vi "TrajectoryExecuteRelative.vi"(8 "Init":bool, 10 "End Relative\nOrientation Deg":dbl, 11 "Trajectory":T1 {"States"."POSE"."ROTATION"."SIN" format="%13.4f"; "States"."POSE"."ROTATION"."COS" format="%13.4f"; "States"."POSE"."ROTATION"."VALUE" format="%13.4f"; "States"."POSE"."TRANSLATION"."Y" format="%14.3f"; "States"."POSE"."TRANSLATION"."X" format="%14.3f"; "TotalTImeSecs" format="%20.3f"}) -> (0 "AtReference":bool, 2 "Done":bool, 3 "Chassis Velocity Target Met,Met,Rad":T6 {"vOmega" format="%10.3f"; "vY" format="%10.3f"; "vX" format="%10.3f"})   [LabVIEW 2023]
uses:
  <vilib>/Rock Robotics/WPI/ThirdParty/JAS_Junk/TrajLib/TypeDef/CHASSIS_SPEEDS.ctl
  <vilib>/Rock Robotics/WPI/ThirdParty/JAS_Junk/TrajLib/TypeDef/TRAJECTORY.ctl
  <vilib>/Rock Robotics/WPI/ThirdParty/JAS_Junk/TrajLib/TypeDef/TRAJ_STATE.ctl
  <vilib>/Rock Robotics/WPI/ThirdParty/JAS_Junk/TrajLib/TypeDef/POSE2D.ctl
  <vilib>/Rock Robotics/WPI/ThirdParty/JAS_Junk/TrajLib/TypeDef/TRANSLATION2D.ctl
  <vilib>/Rock Robotics/WPI/ThirdParty/JAS_Junk/TrajLib/TypeDef/ROTATION2D.ctl
  <vilib>/Rock Robotics/WPI/ThirdParty/JAS_Junk/TrajLib/VI/Util_GetTime_U32.vi
  <vilib>/Rock Robotics/WPI/ThirdParty/JAS_Junk/TrajLib/SwerveOdometry_UpdateX.vi
  <vilib>/Rock Robotics/WPI/ThirdParty/JAS_Junk/TrajLib/SwerveOdometry_ResetPosition.vi
  <vilib>/Rock Robotics/WPI/ThirdParty/JAS_Junk/TrajLib/SwerveOdometry_New.vi
  <vilib>/Rock Robotics/WPI/ThirdParty/JAS_Junk/TrajLib/HolDrvCtrl_New.vi
  <vilib>/Rock Robotics/WPI/ThirdParty/JAS_Junk/TrajLib/HolDrvCtrl_PackPID.vi
  <vilib>/Rock Robotics/WPI/ThirdParty/JAS_Junk/TrajLib/HolDrvCtrl_SetTolerance.vi
  <vilib>/Rock Robotics/WPI/ThirdParty/JAS_Junk/TrajLib/HolDrvCtrl_SetEnabled.vi
  <vilib>/Rock Robotics/WPI/ThirdParty/JAS_Junk/TrajLib/HolDrvCtrl_Calculate_Trajectory.vi
  <vilib>/Rock Robotics/WPI/ThirdParty/JAS_Junk/TrajLib/HolDrvCtrl_AtReference.vi
  <vilib>/Rock Robotics/WPI/ThirdParty/JAS_Junk/TrajLib/ProfiledPIDController_NewPeriod.vi
  <vilib>/Rock Robotics/WPI/ThirdParty/JAS_Junk/TrajLib/ProfiledPIDController_SetIntegratorRange.vi
  <vilib>/Rock Robotics/WPI/ThirdParty/JAS_Junk/TrajLib/ProfiledPIDController_DisableContInput.vi
  <vilib>/Rock Robotics/WPI/ThirdParty/JAS_Junk/TrajLib/ProfiledPIDController_EnableContInput.vi
  <vilib>/Rock Robotics/WPI/ThirdParty/JAS_Junk/TrajLib/TrapProfConstraint_New.vi
  <vilib>/Rock Robotics/WPI/ThirdParty/JAS_Junk/TrajLib/Rotation2d_Plus.vi
  <vilib>/Rock Robotics/WPI/ThirdParty/JAS_Junk/TrajLib/Twist2d_Create.vi
  <vilib>/Rock Robotics/WPI/ThirdParty/JAS_Junk/TrajLib/Rotation2d_Minus.vi
  <vilib>/Rock Robotics/WPI/ThirdParty/JAS_Junk/TrajLib/Pose2d_getTranslation.vi
  <vilib>/Rock Robotics/WPI/ThirdParty/JAS_Junk/TrajLib/Pose2d_New_TRRO.vi
  <vilib>/Rock Robotics/WPI/ThirdParty/JAS_Junk/TrajLib/VI/SwerveModulePosition_Get.vi
  <vilib>/Rock Robotics/WPI/ThirdParty/JAS_Junk/TrajLib/VI/SwerveModulePosition_New.vi
  <vilib>/Rock Robotics/WPI/ThirdParty/JAS_Junk/TrajLib/Twist2d_GetAll.vi
  <vilib>/Rock Robotics/WPI/ThirdParty/JAS_Junk/TrajLib/Pose2d_getRotation.vi
  <vilib>/Rock Robotics/SystemInterfaces/NetworkCommunication/NetComm_UsageReport_report.vi
  <vilib>/Rock Robotics/WPI/ThirdParty/JAS_Junk/TrajLib/PIDController_NewPeriod.vi
  <vilib>/Rock Robotics/WPI/ThirdParty/JAS_Junk/TrajLib/PIDController_SetIntegratorRange.vi
  <vilib>/Rock Robotics/WPI/ThirdParty/JAS_Junk/TrajLib/PIDController_Reset.vi
  <vilib>/Rock Robotics/WPI/ThirdParty/JAS_Junk/TrajLib/HolDrvCtrl_Calculate.vi
  <vilib>/Rock Robotics/WPI/ThirdParty/JAS_Junk/TrajLib/Pose2d_getXYAngle.vi
  <vilib>/Rock Robotics/WPI/ThirdParty/JAS_Junk/TrajLib/Rotation2d_GetRadians.vi
  <vilib>/Rock Robotics/WPI/ThirdParty/JAS_Junk/TrajLib/TrapProfState_New.vi
  <vilib>/Rock Robotics/WPI/ThirdParty/JAS_Junk/TrajLib/PIDController_DisableContinousInput.vi
  <vilib>/Rock Robotics/WPI/ThirdParty/JAS_Junk/TrajLib/PIDController_EnableContinousInput.vi
  <vilib>/Rock Robotics/WPI/ThirdParty/JAS_Junk/TrajLib/Rotation2d_RotateBy.vi
  <vilib>/Rock Robotics/WPI/ThirdParty/JAS_Junk/TrajLib/Rotation2d_UnaryMinus.vi
  <vilib>/Rock Robotics/WPI/ThirdParty/JAS_Junk/TrajLib/Rotation2d_GetAngleCosSin.vi
  <vilib>/Rock Robotics/WPI/ThirdParty/JAS_Junk/TrajLib/Pose2d_RelativeTo.vi
  <vilib>/Rock Robotics/WPI/ThirdParty/JAS_Junk/TrajLib/ProfiledPIDController_Calculate_Meas_Goal.vi
  <vilib>/Rock Robotics/WPI/ThirdParty/JAS_Junk/TrajLib/PIDController_Calculate_SP_PV.vi
  <vilib>/Rock Robotics/WPI/ThirdParty/JAS_Junk/TrajLib/ProfiledPIDController_Reset_PosOnly.vi
  <vilib>/Rock Robotics/WPI/ThirdParty/JAS_Junk/TrajLib/ChassisSpeeds_FromFieldRelativeSpeeds.vi
  <vilib>/Rock Robotics/WPI/ThirdParty/JAS_Junk/TrajLib/Rotation2d_CreateXY.vi
  <vilib>/Rock Robotics/WPI/ThirdParty/JAS_Junk/TrajLib/Transform2d_Create_PosePose.vi
  <vilib>/Rock Robotics/WPI/ThirdParty/JAS_Junk/TrajLib/ProfiledPIDController_SetGoal_PosOnly.vi
  <vilib>/Rock Robotics/WPI/ThirdParty/JAS_Junk/TrajLib/ProfiledPIDController_Calculate_Meas.vi
  <vilib>/Rock Robotics/WPI/ThirdParty/JAS_Junk/TrajLib/PIDController_SetSetpoint.vi
  <vilib>/Rock Robotics/WPI/ThirdParty/JAS_Junk/TrajLib/PIDController_Calculate_PV.vi
  <vilib>/Rock Robotics/WPI/ThirdParty/JAS_Junk/TrajLib/ProfiledPIDController_Reset.vi
  <vilib>/Rock Robotics/WPI/ThirdParty/JAS_Junk/TrajLib/Rotation2d_GetCos.vi
  <vilib>/Rock Robotics/WPI/ThirdParty/JAS_Junk/TrajLib/Rotation2d_GetSin.vi
  <vilib>/Rock Robotics/WPI/ThirdParty/JAS_Junk/TrajLib/Util_CalcDist.vi
  <vilib>/Rock Robotics/WPI/ThirdParty/JAS_Junk/TrajLib/Translation2d_RotateBy.vi
  <vilib>/Rock Robotics/WPI/ThirdParty/JAS_Junk/TrajLib/Translation2d_Minus.vi
  <vilib>/Rock Robotics/WPI/ThirdParty/JAS_Junk/TrajLib/ProfiledPIDController_SetGoal.vi
  <vilib>/Rock Robotics/WPI/ThirdParty/JAS_Junk/TrajLib/TrapProfile_New.vi
  <vilib>/Rock Robotics/WPI/ThirdParty/JAS_Junk/TrajLib/ProfiledPIDController_GetPeriod.vi
  <vilib>/Rock Robotics/WPI/ThirdParty/JAS_Junk/TrajLib/TrapProfile_Calculate.vi
  <vilib>/Rock Robotics/WPI/ThirdParty/JAS_Junk/TrajLib/ControllerUtil_GetModulusError.vi
  <vilib>/Rock Robotics/WPI/ThirdParty/JAS_Junk/TrajLib/Translation2d_Create.vi
  <vilib>/Rock Robotics/WPI/ThirdParty/JAS_Junk/TrajLib/TrapProfile_ShouldFlipAcceleration.vi
  <vilib>/Rock Robotics/WPI/ThirdParty/JAS_Junk/TrajLib/TrapProfile_Direct.vi
  <vilib>/Rock Robotics/WPI/ThirdParty/JAS_Junk/TrajLib/PIDController_GetPeriod.vi
  TrajectoryGlobals.vi
  <vilib>/Rock Robotics/SystemInterfaces/Utilities/FPGA_UtilitiesRead LocalTime.vi
  <vilib>/Rock Robotics/WPI/ThirdParty/JAS_Junk/TrajLib/VI/Util_GetTime_U64.vi
  <vilib>/Rock Robotics/WPI/ThirdParty/JAS_Junk/TrajLib/Globals/Util_LibraryGlobals.vi
  <vilib>/Rock Robotics/WPI/ThirdParty/JAS_Junk/TrajLib/VI/SwerveKinematics_ToTwist2dX.vi
  <vilib>/Rock Robotics/WPI/ThirdParty/JAS_Junk/TrajLib/Pose2d_Exp.vi
  <vilib>/Rock Robotics/WPI/ThirdParty/JAS_Junk/TrajLib/Trajectory_Library.lvlib
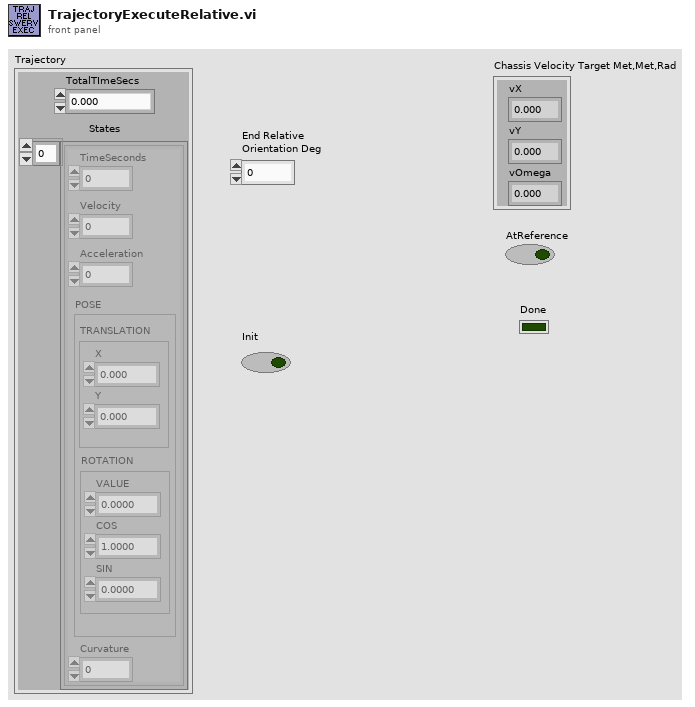
[diagram p1: front panel]
types:
  T1 = typedef "Trajectory_Library.lvlib/TRAJECTORY.ctl" = cluster{"TotalTImeSecs":dbl, "States":T2[]}
  T2 = typedef "Trajectory_Library.lvlib/TRAJ_STATE.ctl" = cluster{"TimeSeconds":dbl, "Velocity":dbl, "Acceleration":dbl, "POSE":T3, "Curvature":dbl}
  T3 = typedef "Trajectory_Library.lvlib/POSE2D.ctl" = cluster{"TRANSLATION":T4, "ROTATION":T5}
  T4 = typedef "Trajectory_Library.lvlib/TRANSLATION2D.ctl" = cluster{"X":dbl, "Y":dbl}
  T5 = typedef "Trajectory_Library.lvlib/ROTATION2D.ctl" = cluster{"VALUE":dbl, "COS":dbl, "SIN":dbl}
  T6 = typedef "Trajectory_Library.lvlib/CHASSIS_SPEEDS.ctl" = cluster{"vX":dbl, "vY":dbl, "vOmega":dbl}
  T7 = typedef "Trajectory_Library.lvlib/SWERVE_DRIVE_MODULE_POSITION.ctl" = cluster{"Distance":dbl, "Angle":T5, "P":bool}
  T8 = typedef "Trajectory_Library.lvlib/SWERVE_DRIVE_KINEMATICS.ctl" = cluster{"NumModules":i32, "InverseKinematics":T9, "ForwardKinematics":T9, "Modules":T4[], "PrevCoR":T4, "SavedModuleStates":T10[]}
  T9 = typedef "NI_Matrix.lvlib/RealMatrix.ctl" = dbl[][]
  T10 = typedef "Trajectory_Library.lvlib/SWERVE_DRIVE_MODULE_STATE.ctl" = cluster{"Speed":dbl, "Angle":T5}
  T11 = typedef "Trajectory_Library.lvlib/PID_TUNING.ctl" = cluster{"Kp":dbl, "Ki":dbl, "Kd":dbl, "MaximumIntegral":dbl, "MinimumIntegral":dbl}
  T12 = typedef "Trajectory_Library.lvlib/PROFILED_PID_CONTROLLER.ctl" = cluster{"Controller":T13, "Goal":T14, "Setpoint":T14, "Constraint":T15}
  T13 = typedef "Trajectory_Library.lvlib/PID_CONTROLLER.ctl" = cluster{"Kp":dbl, "Ki":dbl, "Kd":dbl, "Period":dbl, "Max_Integral":dbl, "Min_Integral":dbl, "Max_Input":dbl, "Min_Input":dbl, "Continuous":bool, "PositionError":dbl, "VelocityError":dbl, "PrevError":dbl, "TotalError":dbl, "PositionTolerance":dbl, "VelocityTolerance":dbl, "SetPoint":dbl, "Kf":dbl, "Prev_Deriv":dbl, "Prev_Deriv 2":dbl, "DerivativeFilter":bool, "Min_Output":dbl, "Max_Output":dbl, "Prev_F_P":dbl, "Prev_F_P_2":dbl, "AntiWindupActive":bool, "Measurement":dbl}
  T14 = typedef "Trajectory_Library.lvlib/TRAPEZOID_PROFILE_STATE.ctl" = cluster{"Position":dbl, "Velocity":dbl}
  T15 = typedef "Trajectory_Library.lvlib/TRAPEZOID_PROFILE_CONSTRAINT.ctl" = cluster{"MaxVelocity":dbl, "MaxAcceleration":dbl}
  T16 = typedef "Trajectory_Library.lvlib/HOLONOMIC_PACK_TUNING.ctl" = cluster{"X PID Tuning":T11, "Y PID Tuning":T11, "thetaProfiledPID_CTRL":T12}
  T17 = typedef "Trajectory_Library.lvlib/HOLONOMIC_DRV_CTRL.ctl" = cluster{"poseTolerance":T3, "poseError":T3, "Enabled":bool, "PID_xCtrl":T13, "PID_yCtrl":T13, "PROF_PID_thetaCtrl":T12, "RotationError":T5, "FirstRun":bool}
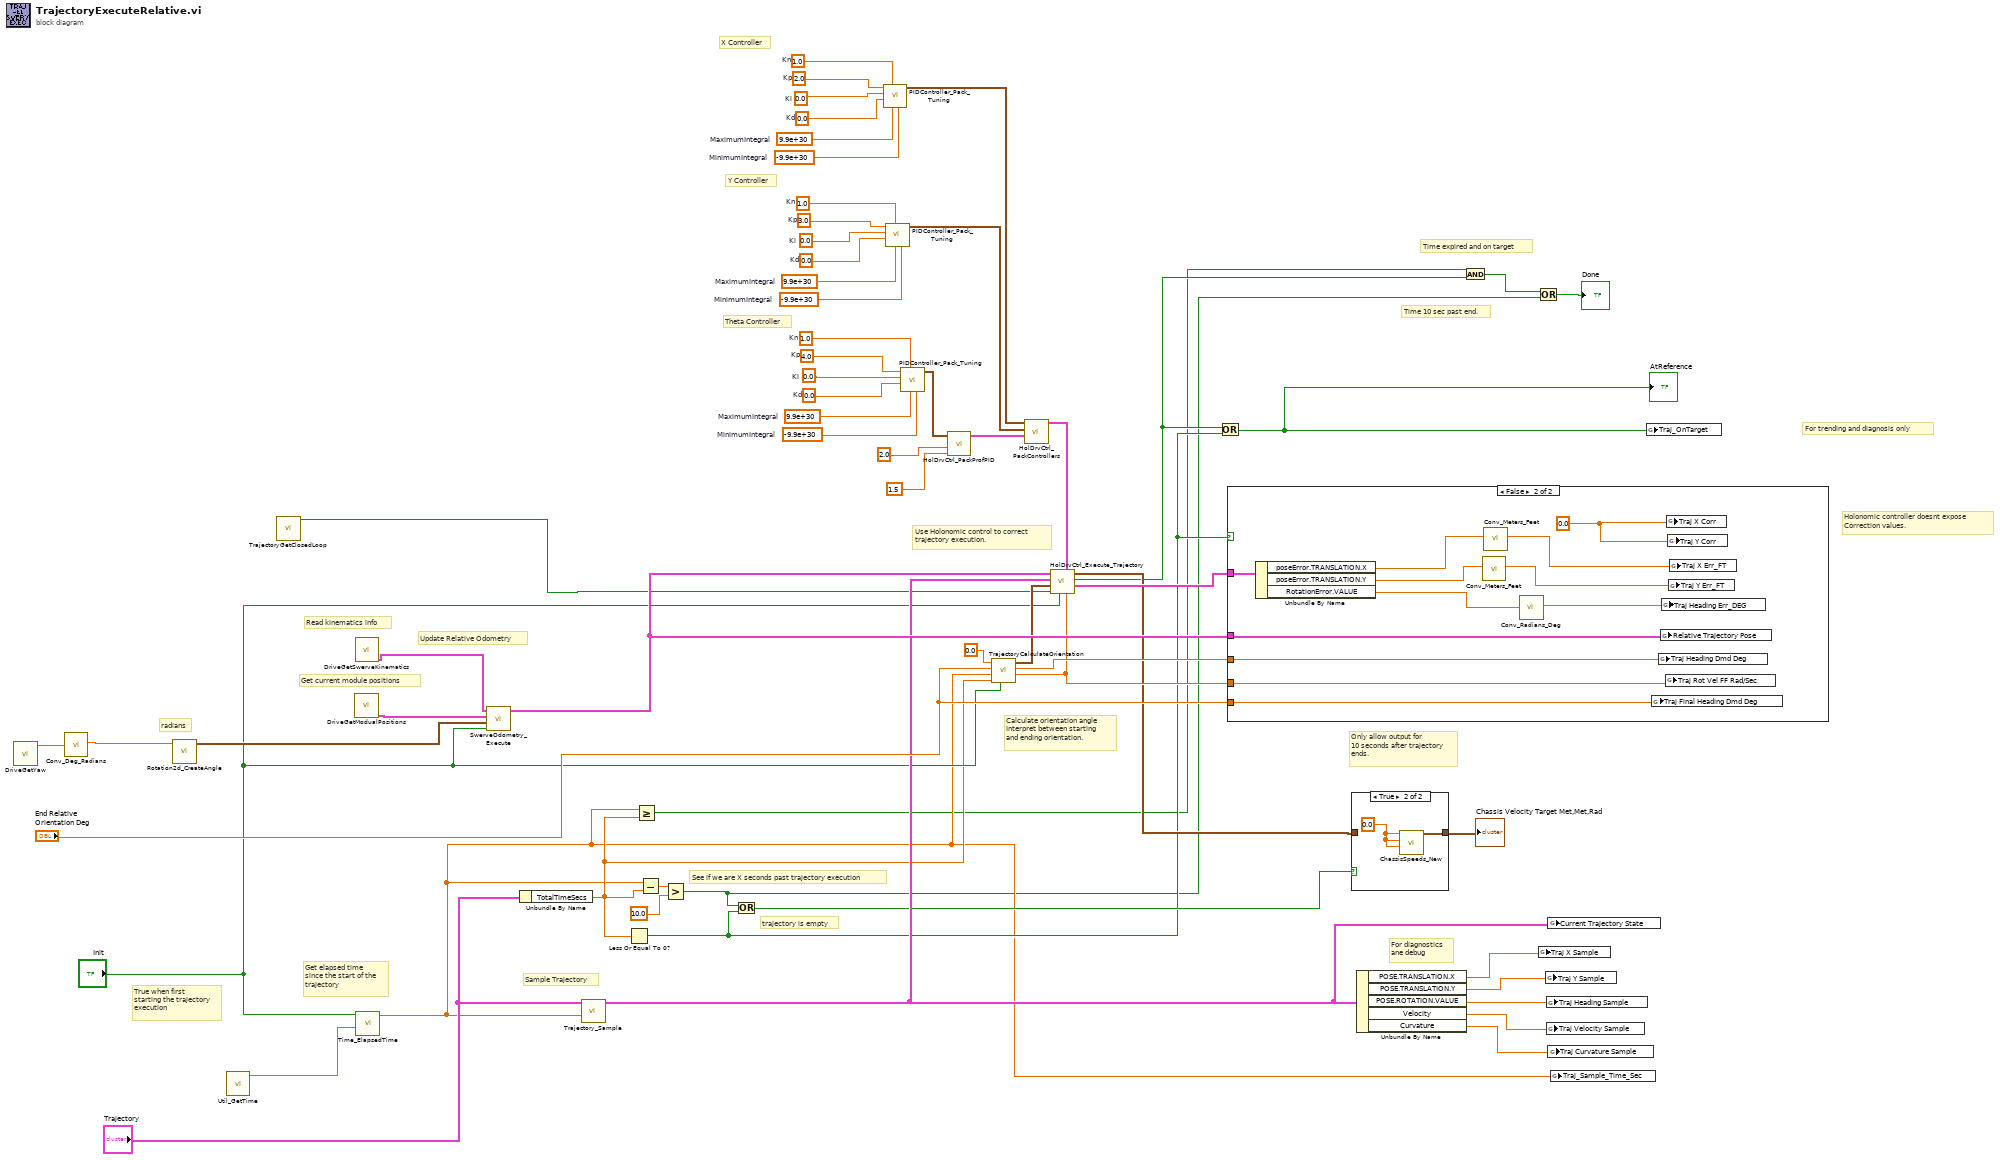
[diagram p0: block diagram]
diagram:
  w30 = 1.0  # Kn
  w33 = 4.0  # Kp
  w42 = 0.0  # Ki
  w43 = 0.0  # Kd
  w44 = 9.9e+30  # MaximumIntegral
  w45 = -9.9e+30  # MinimumIntegral
  w28 = 1.0  # Kn
  w31 = 2.0  # Kp
  w34 = 0.0  # Ki
  w35 = 0.0  # Kd
  w36 = 9.9e+30  # MaximumIntegral
  w37 = -9.9e+30  # MinimumIntegral
  w29 = 1.0  # Kn
  w32 = 3.0  # Kp
  w38 = 0.0  # Ki
  w39 = 0.0  # Kd
  w40 = 9.9e+30  # MaximumIntegral
  w41 = -9.9e+30  # MinimumIntegral
  # "Time 10 sec past end."
  # "Time expired and on target"
  # "trajectory is empty"
  # "Theta Controller"
  # "Y Controller"
  # "X Controller"
  # "Calculate orientation angle\nInterpret between starting\nand ending orientation."
  # "Get current module positions"
  # "True when first\nstarting the trajectory\nexecution"
  # "Get elapsed time\nsince the start of the\ntrajectory"
  # "Holonomic controller doesnt expose\nCorrection values."
  # "Use Holonomic control to correct\ntrajectory execution."
  # "For trending and diagnosis only"
  # "For diagnostics\nane debug"
  # "Update Relative Odometry"
  # "Read kinematics info"
  # "Sample Trajectory"
  # "See if we are X seconds past trajectory execution"
  # "radians"
  # "Only allow output for\n10 seconds after trajectory\nends."
  n1 = call "DriveGetYaw.vi"() -> ("Yaw"=w10:dbl)  [unwired: 11 in]
  n2 = call <vilib>:"Conv_Deg_Radians.vi"("Degress"=w10) -> ("Radians"=w9:dbl)  [unwired: 10 in]
  n3 = call <vilib>:"Rotation2d_CreateAngle.vi"("Angle"=w9) -> ("ROTATION"=w58:T5)  [unwired: 10 in]
  n4 = call <vilib>:"Util_GetTime.vi"() -> ("FPGA_Time_Seconds"=w57:dbl)  [unwired: 9 in, 2 out]
  n5 = call "TrajectoryGetClosedLoop.vi"() -> ("AUTO_CLOSED_LOOP"=w15:bool)  [unwired: 11 in]
  n6 = call "DriveGetModualPositions.vi"() -> ("Swerve_Drive_Modual_Positions"=w13:T7[])  [unwired: 11 in]
  n7 = call "DriveGetSwerveKinematics.vi"() -> ("SWERVE_DRIVE_KINEMATICS"=w14:T8)  [unwired: 11 in]
  n8 = call <vilib>:"Time_ElapsedTime.vi"("PassthroughTime_SEC"=w57, "Reset"="Init") -> ("Elapsed Time Sec"=w6:dbl)  [unwired: 9 in]
  n9 = call <vilib>:"SwerveOdometry_Execute.vi"("Init"="Init", "Rotation"=w58, "Swerve Module Positions"=w13, "SWERVE_DRIVE_KINEMATICS"=w14) -> ("Current Pose"=w26:T3)  [unwired: 5 in, 2 out]
  n10 = Unbundle By Name("Trajectory") -> ("TotalTImeSecs"=w7:dbl)
  n11 = call <vilib>:"Trajectory_Sample.vi"("Time"=w6, "InputTRAJECTORY"="Trajectory") -> ("OutputTRAJ_STATE"=w21:T2)  [unwired: 9 in]
  n12 = Less Or Equal To 0?(x=w7) -> (x <= 0?=w17:bool)
  n13 = Greater Or Equal?(x=w6, y=w7) -> (x >= y?=w2:bool)
  n14 = Subtract(x=w6, y=w7) -> (x-y=w61:dbl)
  n15 = Greater?(x=w61, y=10.0) -> (0:w1:bool)
  n16 = Or(x=w1, y=w17) -> (x .or. y?=w19:bool)
  n17 = call <vilib>:"PIDController_Pack_Tuning.vi"("MinimumIntegral"=w37, "MaximumIntegral"=w36, "Kn"=w28, "Kd"=w35, "Ki"=w34, "Kp"=w31) -> ("PID Tuning"=w46:T11)  [unwired: 5 in]
  n18 = call <vilib>:"PIDController_Pack_Tuning.vi"("MinimumIntegral"=w41, "MaximumIntegral"=w40, "Kn"=w29, "Kd"=w39, "Ki"=w38, "Kp"=w32) -> ("PID Tuning"=w47:T11)  [unwired: 5 in]
  n19 = call <vilib>:"PIDController_Pack_Tuning.vi"("MinimumIntegral"=w45, "MaximumIntegral"=w44, "Kn"=w30, "Kd"=w43, "Ki"=w42, "Kp"=w33) -> ("PID Tuning"=w27:T11)  [unwired: 5 in]
  n20 = call <vilib>:"HolDrvCtrl_PackProfPID.vi"("Max Accel"=1.5, "Max Speed"=2.0, "Theta PID Tuning"=w27) -> ("Theta PID CONTROLLER"=w48:T12)  [unwired: 8 in]
  n21 = call "TrajectoryCalculateOrientation.vi"("Init"="Init", "Total Trajectory Time Sec"=w7, "Elapsed Traj Time Sec"=w6, "End Orientation Demand DEG"="End Relative\nOrientation Deg", "Starting Orientation  DEG"=0.0) -> ("Rotational Velocity Rad Per Sec"=w23:dbl, "Orientation Demand Deg"=w51:dbl, "Orientation Demand"=w25:T5)  [unwired: 4 in]
  n22 = call <vilib>:"HolDrvCtrl_PackControllers.vi"("thetaProfiledPID_CTRL"=w48, "Y PID Tuning"=w47, "X PID Tuning"=w46) -> ("HOLONOMIC_CTRL_PACK_TUNING"=w49:T16)  [unwired: 8 in]
  n23 = call <vilib>:"HolDrvCtrl_Execute_Trajectory.vi"("Rotational Velocity Feedforward \nRad/Sec"=w23, "HOLONOMIC_CTRL_PACK_TUNING"=w49, "Reset"="Init", "Enable"=w15, "angleRef"=w25, "desiredTrajState"=w21, "currentPose"=w26) -> ("outHOLONOMIC_DRV_CTRL"=w24:T17, "AtReference"=w3:bool, "calcChassisSpeed"=w20:T6)  [unwired: 2 in]
  n24 = Or(x=w3, y=w17) -> (x .or. y?=w18:bool)
  "AtReference" <- w18
  n25 = case shown="False" w17 {
    tunnel: w51 -> [_ w72]
    tunnel: "End Relative\nOrientation Deg" -> [_ w71]
    tunnel: w26 -> [_ w65]
    tunnel: w24 -> [_ w64]
    tunnel: w23 -> [_ w63]
    frame True {
    }
    frame False {
      w73 = 0.0 ("Y Corr")
      n26 = Unbundle By Name(w64) -> ("poseError.TRANSLATION.X"=w69:dbl, "poseError.TRANSLATION.Y"=w68:dbl, "RotationError.VALUE"=w62:dbl)
      n27 = call <vilib>:"Conv_Meters_Feet.vi"("Meters"=w68) -> ("Feet"=w67:dbl)  [unwired: 10 in]
      n28 = call <vilib>:"Conv_Meters_Feet.vi"("Meters"=w69) -> ("Feet"=w66:dbl)  [unwired: 10 in]
      n29 = call <vilib>:"Conv_Radians_Deg.vi"("Radians"=w62) -> ("Degrees"=w70:dbl)  [unwired: 10 in]
      n30 = global write "TrajectoryGlobals.vi" "Traj Final Heading Dmd Deg"(w71) -> ()
      n31 = global write "TrajectoryGlobals.vi" "Traj Heading Dmd Deg"(w72) -> ()
      n32 = global write "TrajectoryGlobals.vi" "Relative Trajectory Pose"(w65) -> ()
      n33 = global write "TrajectoryGlobals.vi" "Traj Heading Err_DEG"(w70) -> ()
      n34 = global write "TrajectoryGlobals.vi" "Traj Rot Vel FF Rad/Sec"(w63) -> ()
      n35 = global write "TrajectoryGlobals.vi" "Traj X Corr"(w73) -> ()
      n36 = global write "TrajectoryGlobals.vi" "Traj Y Corr"(w73) -> ()
      n37 = global write "TrajectoryGlobals.vi" "Traj Y Err_FT"(w67) -> ()
      n38 = global write "TrajectoryGlobals.vi" "Traj X Err_FT"(w66) -> ()
    }
  }
  n39 = case shown="True" w19 {
    tunnel: w20 -> [w74 _]
    tunnel: [w74 w75] -> w59
    frame False {
    }
    frame True {
      w76 = 0.0 ("vX")
      n40 = call <vilib>:"ChassisSpeeds_New.vi"("vAngular"=w76, "vY"=w76, "vX"=w76) -> ("CHASSIS"=w75:T6)  [unwired: 8 in]
    }
  }
  "Chassis Velocity Target Met,Met,Rad" <- w59
  n41 = Unbundle By Name(w21) -> ("POSE.TRANSLATION.X"=w56:dbl, "POSE.TRANSLATION.Y"=w55:dbl, "POSE.ROTATION.VALUE"=w54:dbl, "Velocity"=w53:dbl, "Curvature"=w52:dbl)
  n42 = And(x=w2, y=w3) -> (x .and. y?=w5:bool)
  n43 = Or(x=w5, y=w1) -> (x .or. y?=→"Done":bool)
  n44 = global write "TrajectoryGlobals.vi" "Traj X Sample"(w56) -> ()
  n45 = global write "TrajectoryGlobals.vi" "Traj Y Sample"(w55) -> ()
  n46 = global write "TrajectoryGlobals.vi" "Traj Heading Sample"(w54) -> ()
  n47 = global write "TrajectoryGlobals.vi" "Traj Velocity Sample"(w53) -> ()
  n48 = global write "TrajectoryGlobals.vi" "Current Trajectory State"(w21) -> ()
  n49 = global write "TrajectoryGlobals.vi" "Traj Curvature Sample"(w52) -> ()
  n50 = global write "TrajectoryGlobals.vi" "Traj_Sample_Time_Sec"(w6) -> ()
  n51 = global write "TrajectoryGlobals.vi" "Traj_OnTarget"(w18) -> ()
